vi "Network Functions (avg).vi"(8 "dt":dbl=1.0 format="%0.6p", 10 "Response Signal":dbl[][](array[numeric]), 11 "Stimulus Signal":dbl[][](array[numeric])) -> (0 "df":dbl format="%0.2f", 1 "Impulse Response (avg)":dbl[](array[numeric]), 2 "Coherence Function (0..1)":dbl[](array[numeric]), 3 "Frequency Response (avg)":T2 {"Phase (radians)" format="%.2f"; "Magnitude (Gain)" format="%.2f"}, 5 "Cross Power Spectrum (avg)":T1 {"Phase (radians)" format="%.2f"; "Magnitude (Vrms^2)" format="%.2f"})   [LabVIEW 2020, in "NI_AALPro.lvlib"]
doc: "Computes the single-sided <B>Coherence Function</B>, the averaged single-sided <B>Cross Power Spectrum</B>, the averaged single-sided <B>Frequency Response</B>, or transfer function, and the <B>Impulse Response</B>."
uses:
  <vilib>/Analysis/NI_AALPro.lvlib
  <vilib>/Analysis/2dsp.llb/Power Spectrum (DBL).vi
  <vilib>/Analysis/2dsp.llb/Cross Power (DBL).vi
panel:
  # "Network Functions"
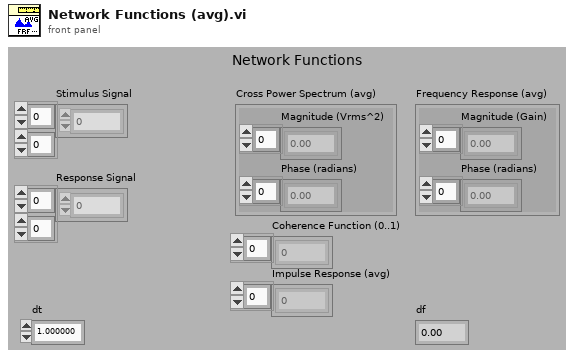
[diagram p1: front panel]
types:
  T1 = cluster{"Magnitude (Vrms^2)":dbl[], "Phase (radians)":dbl[]}
  T2 = cluster{"Magnitude (Gain)":dbl[], "Phase (radians)":dbl[]}
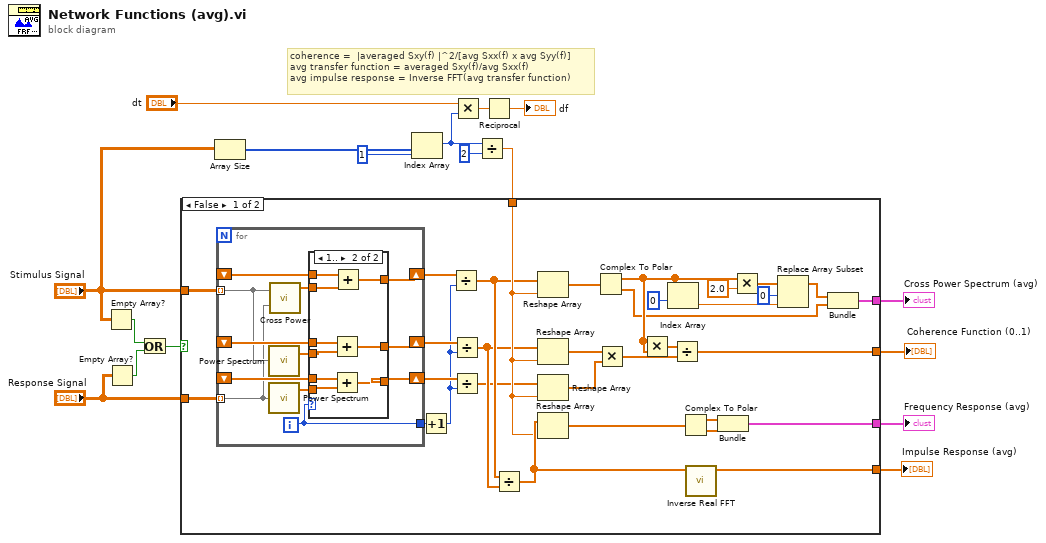
[diagram p0: block diagram]
diagram:
  # "coherence =  |averaged Sxy(f) |^2/[avg Sxx(f) x avg Syy(f)]\navg transfer function = averaged Sxy(f)/avg Sxx(f)\navg impulse response = Inverse FFT(avg transfer function)"
  n1 = Empty Array?(array="Stimulus Signal") -> (empty?=w3:bool)
  n2 = Empty Array?(array="Response Signal") -> (empty?=w2:bool)
  n3 = Or(x=w3, y=w2) -> (x .or. y?=w1:bool)
  n4 = Array Size(array="Stimulus Signal") -> (size(s)=w15:i32[])
  n5 = Index Array(array=w15, index=1) -> (element=w9:i32)
  n6 = Multiply(x="dt", y=w9) -> (x*y=w16:dbl)
  n7 = Divide(x=w9, y=2) -> (x/y=w11:dbl)
  n8 = case shown="False" w1 {
    tunnel: [w44 _] -> w12
    tunnel: w11 -> [w39 _]
    tunnel: [w30 _] -> w10
    tunnel: "Response Signal" -> [w21 _]
    tunnel: "Stimulus Signal" -> [w20 _]
    tunnel: [w19 _] -> w7
    tunnel: [w18 _] -> w6
    frame False {
      n9 = for {
        tunnel: w21 -> [w50] mode=indexing
        shift-right: [w55] -> w48
        shift-left: _ -> [w56]
        shift-right: [w59] -> w49
        shift-left: _ -> [w58]
        tunnel: [w61] -> w47
        tunnel: w20 -> [w51] mode=indexing
        shift-right: [w53] -> w46
        shift-left: _ -> [w54]
        i -> [w61]
        n10 = call-poly <vilib>:"Power Spectrum.vi"("X"=w51) -> ("Power Spectrum"=w60:dbl[])  [unwired: 1 out]
        n11 = call-poly <vilib>:"Power Spectrum.vi"("X"=w50) -> ("Power Spectrum"=w57:dbl[])  [unwired: 1 out]
        n12 = call-poly <vilib>:"Cross Power.vi"("Y"=w50, "X"=w51) -> ("Sxy"=w52:cdb[])  [unwired: 1 out]
        n13 = case shown="1.." w61 {
          tunnel: w60 -> [w64 w73]
          tunnel: [w64 w71] -> w59
          tunnel: w58 -> [_ w72]
          tunnel: w57 -> [w63 w69]
          tunnel: w56 -> [_ w70]
          tunnel: [w63 w68] -> w55
          tunnel: w52 -> [w62 w66]
          tunnel: [w62 w67] -> w53
          tunnel: w54 -> [_ w65]
          frame ..0 {
          }
          frame 1.. {
            n14 = Add(x=w72, y=w73) -> (x+y=w71:dbl[])
            n15 = Add(x=w70, y=w69) -> (x+y=w68:dbl[])
            n16 = Add(x=w65, y=w66) -> (x+y=w67:cdb[])
          }
        }
      }
      n17 = Increment(x=w47) -> (x+1=w45:i32)
      n18 = Divide(x=w46, y=w45) -> (x/y=w26:cdb[])
      n19 = Divide(x=w49, y=w45) -> (x/y=w25:dbl[])
      n20 = Divide(x=w48, y=w45) -> (x/y=w22:dbl[])
      n21 = Divide(x=w26, y=w25) -> (x/y=w40:cdb[])
      n22 = Reshape Array(w26, w39) -> (w27:cdb[])
      n23 = Reshape Array(w25, w39) -> (w24:dbl[])
      n24 = Reshape Array(w22, w39) -> (w23:dbl[])
      n25 = Reshape Array(w40, w39) -> (w41:cdb[])
      n26 = Complex To Polar(r * e^(i*theta)=w27) -> (r=w35:dbl[], theta=w28:dbl[])
      n27 = Multiply(x=w24, y=w23) -> (x*y=w37:dbl[])
      n28 = Multiply(x=w35, y=w35) -> (x*y=w38:dbl[])
      n29 = Index Array(array=w35, index=0) -> (element=w31:dbl)
      n30 = Divide(x=w38, y=w37) -> (x/y=w30:dbl[])
      n31 = Complex To Polar(r * e^(i*theta)=w41) -> (r=w43:dbl[], theta=w42:dbl[])
      n32 = call <vilib>:"Inverse Real FFT.vi"("FFT {X}"=w40) -> ("X"=w44:dbl[])  [unwired: 9 in, 1 out]
      n33 = Bundle(w43, w42) -> (w19:cluster{dbl[], dbl[]})  [unwired: 1 in]
      n34 = Multiply(x=w35, y=2.0) -> (x*y=w33:dbl[])
      n35 = Replace Array Subset(array=w33, new element=w31, index=0) -> (w29:dbl[])
      n36 = Bundle(w29, w28) -> (w18:cluster{dbl[], dbl[]})  [unwired: 1 in]
    }
    frame True {
    }
  }
  "Coherence Function (0..1)" <- w10
  "Impulse Response (avg)" <- w12
  "Frequency Response (avg)" <- w7
  "Cross Power Spectrum (avg)" <- w6
  n37 = Reciprocal(x=w16) -> (1/x=→"df":dbl)
